vi "PicoScope5000aPowerSource.vi"(6 "USB 3.0 on non-USB 3.0 port control":bool=TRUE, 8 "USB Powered control":bool=TRUE, 9 "handle in":i16, 10 "PICO STATUS IN":u32 format="%#.0f", 11 "error in (no error)":errorcluster) -> (0 "USB Powered":bool=TRUE, 1 "handle out":i16, 2 "PICO STATUS OUT":u32, 3 "error out":errorcluster, 4 "USB 3.0 on non-USB 3.0 Port":bool=TRUE)   [LabVIEW 2020]
uses:
  ps5000a.dll
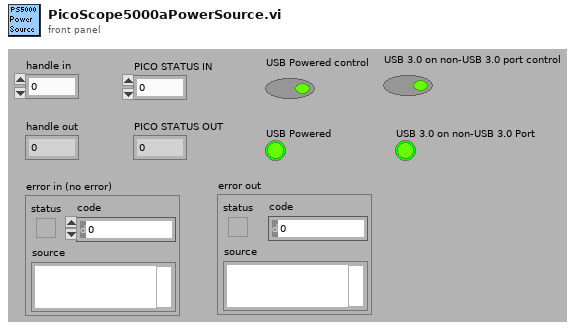
[diagram p1: front panel]
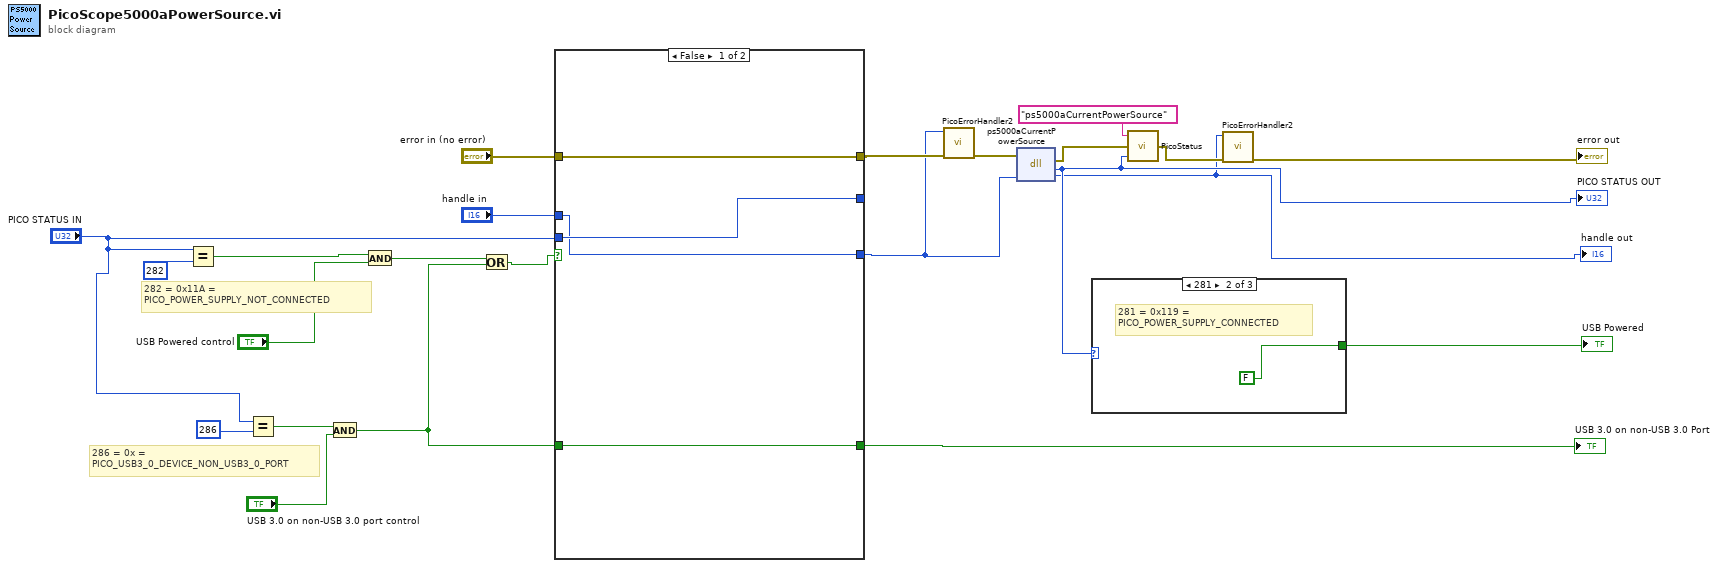
[diagram p0: block diagram]
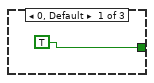
[diagram p2: hidden frame]
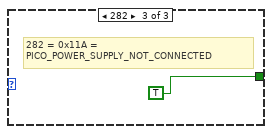
[diagram p3: hidden frame]
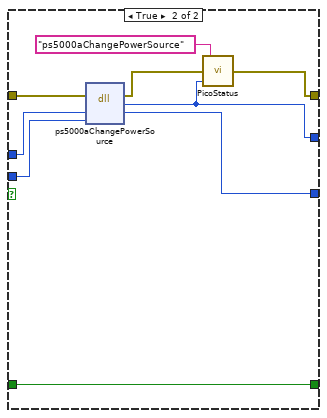
[diagram p4: hidden frame]
diagram:
  # "286 = 0x = \nPICO_USB3_0_DEVICE_NON_USB3_0_PORT"
  # "282 = 0x11A = \nPICO_POWER_SUPPLY_NOT_CONNECTED"
  n1 = Equal?(x="PICO STATUS IN", y=u32 282) -> (x = y?=w22:bool)
  n2 = Equal?(x="PICO STATUS IN", y=u32 286) -> (x = y?=w18:bool)
  n3 = And(x=w18, y="USB 3.0 on non-USB 3.0 port control") -> (x .and. y?=w1:bool)
  n4 = And(x=w22, y="USB Powered control") -> (x .and. y?=w15:bool)
  n5 = Or(x=w15, y=w1) -> (x .or. y?=w14:bool)
  n6 = case shown="False" w14 {
    tunnel: "PICO STATUS IN" -> [w27 w35]
    tunnel: [w27 w28] -> _
    tunnel: [w26 w30] -> w6
    tunnel: "error in (no error)" -> [w26 w36]
    tunnel: "handle in" -> [w25 w34]
    tunnel: [w25 w33] -> w5
    tunnel: w1 -> [w24 w32]
    tunnel: [w24 w32] -> w12
    frame False {
    }
    frame True {
      n7 = dll-call lib="ps5000a.dll" fn="ps5000aChangePowerSource"(error in=w36, "handle"=w34, "powerSource"=w35) -> (error out=w29:errorcluster, "PICO_STATUS"=w28:u32, "handle"=w33:i16)  [unwired: 3 in, 1 out]
      n8 = call "PicoStatus.vi"("PICO STATUS"=w28, "error in"=w29, "source"="ps5000aChangePowerSource") -> ("error out"=w30:errorcluster)
    }
  }
  "USB 3.0 on non-USB 3.0 Port" <- w12
  n9 = call "PicoErrorHandler2.vi"("error in (no error)"=w6, "handle In"=w5) -> ("error out"=w10:errorcluster)  [unwired: 9 in]
  n10 = dll-call lib="ps5000a.dll" fn="ps5000aCurrentPowerSource"(error in=w10, "handle"=w5) -> (error out=w9:errorcluster, "PICO_STATUS"=w4:u32, "handle"=w3:i16)  [unwired: 2 in, 1 out]
  "PICO STATUS OUT" <- w4
  "handle out" <- w3
  n11 = case shown="281" w4 {
    tunnel: [TRUE FALSE TRUE] -> w2
    frame 0, Default {
    }
    frame 281 {
      # "281 = 0x119 = \nPICO_POWER_SUPPLY_CONNECTED"
    }
    frame 282 {
      # "282 = 0x11A = \nPICO_POWER_SUPPLY_NOT_CONNECTED"
    }
  }
  "USB Powered" <- w2
  n12 = call "PicoStatus.vi"("PICO STATUS"=w4, "error in"=w9, "source"="ps5000aCurrentPowerSource") -> ("error out"=w8:errorcluster)
  n13 = call "PicoErrorHandler2.vi"("error in (no error)"=w8, "handle In"=w3) -> ("error out"=→"error out":errorcluster)  [unwired: 9 in]
